vi "Hat Switch Interpreter.vi"(5 "JoystickDevRef":T1) -> (0 "Buttons":bool[](array[boolean]), 1 "Buttons Pressed":bool[](array[boolean]), 2 "Enum Status":T4(ring), 3 "Numeric Status":u8, 4 "Hat Switch Cluster":T3)   [LabVIEW 2013]
uses:
  <vilib>/Rock Robotics/WPI/Joystick/WPI_JoystickDevRef.ctl
  <vilib>/Rock Robotics/WPI/Joystick/WPI_JoystickDeviceEnum.ctl
panel:
  # "ENUM LAYOUT"
  # "NUMERIC LAYOUT"
  # "North"
  # "1"
  # "Northeast"
  # "2"
  # "Northwest"
  # "8"
  # "West"
  # "East"
  # "7"
  # "3"
  # "Null"
  # "0"
  # "Southwest"
  # "Southeast"
  # "6"
  # "4"
  # "5"
  # "South"
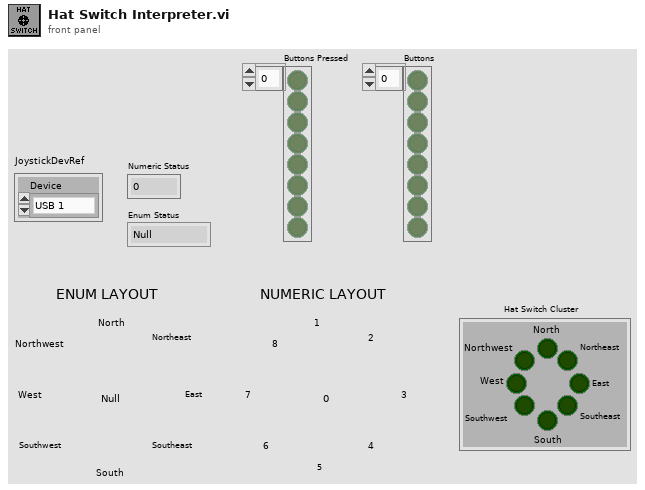
[diagram p1: front panel]
types:
  T1 = typedef "WPI_JoystickDevRef.ctl" = cluster{"Device":T2}
  T2 = typedef "WPI_JoystickDeviceEnum.ctl" = enum16{"USB 1", "USB 2", "USB 3", "USB 4", "Kinect 1", "Kinect 2"}
  T3 = cluster{"North":bool, "Northeast":bool, "East":bool, "Southeast":bool, "South":bool, "Southwest":bool, "West":bool, "Northwest":bool}
  T4 = enum8{"Null", "North", "Northeast", "East", "Southeast", "South", "Southwest", "West", "Northwest"}
  T5 = cluster{"North":bool, "Northeast":bool, "East":bool, "Southeast":bool, "South":bool, "Northwest":bool, "Southwest":bool, "West":bool}
  T6 = cluster{"axis 1 (x)":dbl, "axis 2 (y)":dbl, "axis 3 (throttle)":dbl, "axis 4":dbl, "axis 5":dbl, "axis 6":dbl}
  T7 = cluster{"[0]":bool, "[1]":bool, "[2]":bool, "[3]":bool, "[4]":bool, "[5]":bool, "[6]":bool, "[7]":bool, "[8]":bool}
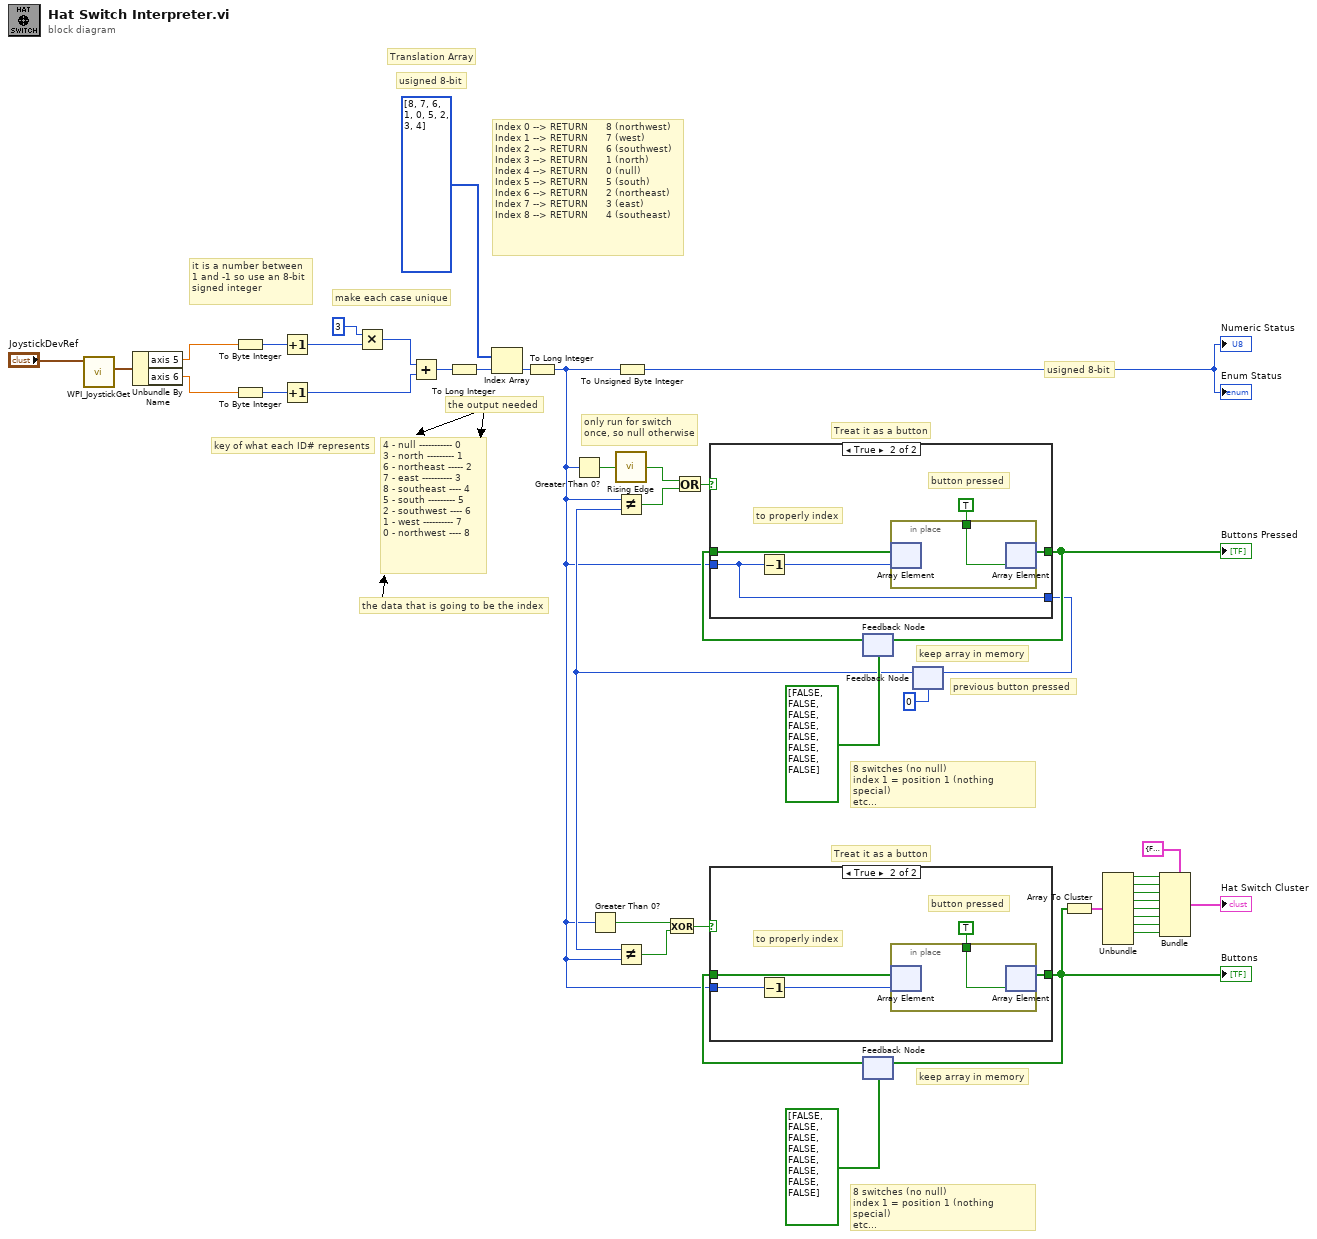
[diagram p0: block diagram]
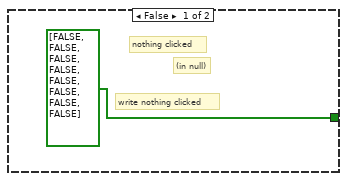
[diagram p2: hidden frame]
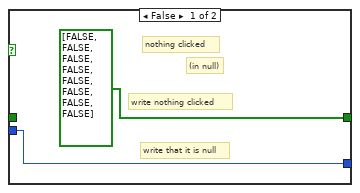
[diagram p3: hidden frame]
diagram:
  # "keep array in memory"
  # "8 switches (no null)\nindex 1 = position 1 (nothing special)\netc..."
  # "Treat it as a button"
  # "only run for switch\nonce, so null otherwise"
  # "keep array in memory"
  # "previous button pressed"
  # "8 switches (no null)\nindex 1 = position 1 (nothing special)\netc..."
  # "Treat it as a button"
  # "usigned 8-bit"
  # "the data that is going to be the index"
  # "the output needed"
  # "key of what each ID# represents"
  # "Index 0 --> RETURN      8 (northwest)\nIndex 1 --> RETURN      7 (west)\nIndex 2 --> RETURN      6 (southwest)\nIndex 3 --> RETURN      1 (north)\nIndex 4 --> RETURN      0 (null)\nIndex 5 --> RETURN      5 (south)\nIndex 6 --> RETURN      2 (northeast)\nIndex 7 --> RETURN      3 (east)\nIndex 8 --> RETURN      4 (southeast)"
  # "4 - null ----------- 0\n3 - north --------- 1\n6 - northeast ----- 2\n7 - east ---------- 3\n8 - southeast ---- 4\n5 - south --------- 5\n2 - southwest ---- 6\n1 - west ---------- 7\n0 - northwest ---- 8"
  # "Translation Array"
  # "usigned 8-bit"
  # "it is a number between\n1 and -1 so use an 8-bit\nsigned integer"
  # "make each case unique"
  n1 = call <vilib>:"WPI_JoystickGet.vi"("JoystickDevRef"="JoystickDevRef") -> ("Axes"=w3:T6)  [unwired: 4 in, 2 out]
  n2 = Unbundle By Name(w3) -> ("axis 5"=w2:dbl, "axis 6"=w1:dbl)
  n3 = To Byte Integer(number=w2) -> (8bit integer=w39:i8)
  n4 = To Byte Integer(number=w1) -> (8bit integer=w38:i8)
  n5 = Increment(x=w39) -> (x+1=w43:i8)
  n6 = Increment(x=w38) -> (x+1=w40:i8)
  n7 = Multiply(x=i8 3, y=w43) -> (x*y=w41:i8)
  n8 = Add(x=w41, y=w40) -> (x+y=w36:i8)
  n9 = To Long Integer(number=w36) -> (32bit integer=w35:i32)
  n10 = Index Array(array=u8[] [8, 7, 6, 1, 0, 5, 2, 3, 4], index=w35) -> (element=w26:u8)
  n11 = To Long Integer(number=w26) -> (32bit integer=w19:i32)
  n12 = Greater Than 0?(x=w19) -> (x > 0?=w29:bool)
  n13 = Greater Than 0?(x=w19) -> (x > 0?=w21:bool)
  n14 = call "Rising Edge.vi"("Input"=w29) -> ("Rising Edge"=w28:bool)
  n15 = To Unsigned Byte Integer(number=w19) -> (unsigned 8bit integer=→"Numeric Status" →"Enum Status":u8)
  n16 = feedback #1(bool[] [FALSE, FALSE, FALSE, FALSE, FALSE, FALSE, FALSE, FALSE]) -> (w33:bool[])
  n17 = feedback #2(bool[] [FALSE, FALSE, FALSE, FALSE, FALSE, FALSE, FALSE, FALSE]) -> (w23:bool[])
  n18 = feedback #3(0) -> (w20:i32)
  n19 = Not Equal?(x=w19, y=w20) -> (x != y?=w25:bool)
  n20 = Not Equal?(x=w20, y=w19) -> (x != y?=w17:bool)
  n21 = Exclusive Or(1:w17, 2:w21) -> (0:w18:bool)
  n22 = Or(x=w28, y=w25) -> (x .or. y?=w27:bool)
  n23 = case shown="True" w27 {
    tunnel: w33 -> [_ w50]
    tunnel: [bool[] [FALSE, FALSE, FALSE, FALSE, FALSE, FALSE, FALSE, FALSE] w49] -> w32
    tunnel: w19 -> [w45 w46]
    tunnel: [w45 w46] -> w30
    frame False {
      # "write nothing clicked"
      # "write that it is null"
      # "(in null)"
      # "nothing clicked"
    }
    frame True {
      # "to properly index"
      # "button pressed"
      n24 = Decrement(x=w46) -> (x-1=w47:i32)
      n25 = in-place {
        in-place-border: TRUE -> [w51]
        n26 = in-place-array #4(w50, w47) -> ()  [unwired: 1 out]
        n27 = in-place-array #4(w51) -> (w49:bool[])  [unwired: 1 out]
      }
    }
  }
  "Buttons Pressed" <- w32
  n28 = case shown="True" w18 {
    tunnel: w23 -> [_ w57]
    tunnel: [bool[] [FALSE, FALSE, FALSE, FALSE, FALSE, FALSE, FALSE, FALSE] w56] -> w16
    tunnel: w19 -> [_ w53]
    frame False {
      # "write nothing clicked"
      # "(in null)"
      # "nothing clicked"
    }
    frame True {
      # "to properly index"
      # "button pressed"
      n29 = Decrement(x=w53) -> (x-1=w54:i32)
      n30 = in-place {
        in-place-border: TRUE -> [w58]
        n31 = in-place-array #5(w57, w54) -> ()  [unwired: 1 out]
        n32 = in-place-array #5(w58) -> (w56:bool[])  [unwired: 1 out]
      }
    }
  }
  "Buttons" <- w16
  n33 = feedback-in #1(w32) -> ()
  n34 = feedback-in #2(w16) -> ()
  n35 = feedback-in #3(w30) -> ()
  n36 = Array To Cluster(array=w16) -> (cluster=w15:T7)
  n37 = Unbundle(w15) -> ("[0]"=w13:bool, "[1]"=w5:bool, "[2]"=w6:bool, "[3]"=w7:bool, "[4]"=w8:bool, "[5]"=w9:bool, "[6]"=w10:bool, "[7]"=w11:bool)  [unwired: 1 out]
  n38 = Bundle(cluster=T5 {"North"=FALSE, "Northeast"=FALSE, "East"=FALSE, "Southeast"=FALSE, "South"=FALSE, "Northwest"=FALSE, "Southwest"=FALSE, "West"=FALSE} ("Hat Switch Cluster"), "North"=w13, "Northeast"=w5, "East"=w6, "Southeast"=w7, "South"=w8, "Northwest"=w9, "Southwest"=w10, "West"=w11) -> (→"Hat Switch Cluster":T5)
